vi "simple_calculator.vi"() -> ()   [LabVIEW 2021]
panel:
  out "a / b =":sgl format="%#.2f"
  out "a - b =":i32
  out "a+ b =":i32
  out "a * b =":i32
  in  "?":bool
  in  "?":bool
  in  "b":i32=5
  in  "a":i32=10
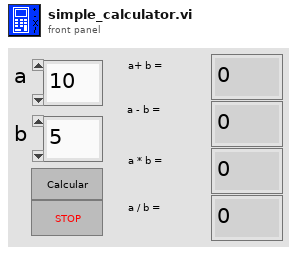
[diagram p1: front panel]
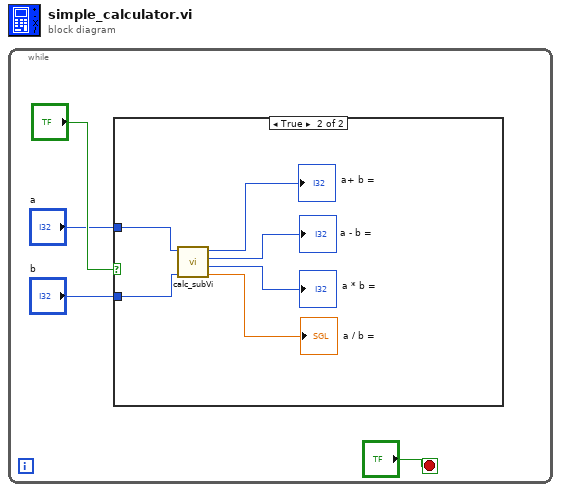
[diagram p0: block diagram]
diagram:
  n1 = while {
    stop <- "?" stop-if-true
    n2 = case shown="True" "?" {
      tunnel: "b" -> [_ w5]
      tunnel: "a" -> [_ w10]
      frame False {
      }
      frame True {
        n3 = call "calc_subVi.vi"("b"=w5, "a"=w10) -> ("Division"=→"a / b =":sgl, "Multiplication"=→"a * b =":i32, "Subtract"=→"a - b =":i32, "Sum"=→"a+ b =":i32)  [unwired: 6 in]
      }
    }
  }
